vi "Log_MessageHandler_AddMessageToLog.vi"(7 "EVE reference in":refnum<data-value>, 8 "error in (no error)":errorcluster, 10 "Messages.lvclass":refnum<class "Messages.lvclass">, 11 "MessageHandler.lvclass in":refnum<class "MessageHandler.lvclass">) -> (0 "error out":errorcluster, 3 "MessageHandler.lvclass out":refnum<class "MessageHandler.lvclass">)   [LabVIEW 2013, in "MessageHandler.lvclass"]
uses:
  Class/MessageHandler.lvclass
  001 - MAIN/Class/Messages/Messages.lvclass
  001 - MAIN/Class/EVE/EVE.lvclass
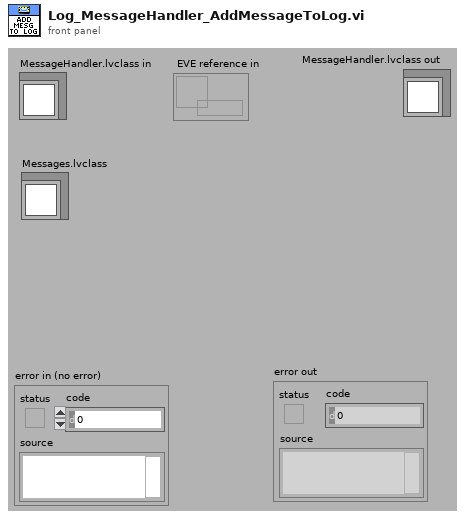
[diagram p1: front panel]
types:
  T1 = typedef "EVE.lvclass/App_GenericSettings.ctl" = cluster{"SpecificSettings":cluster{"FolderPath":path, "XMLFile":string}, "Log":cluster{"MaxLogFiles":i32, "MaxLogMessagesPerFile":i32}, "Debug":cluster{"Active":bool}, "Dictionnary":cluster{"FolderPath":path, "TradFile":string}, "Ressources":cluster{"FolderPath":path}}
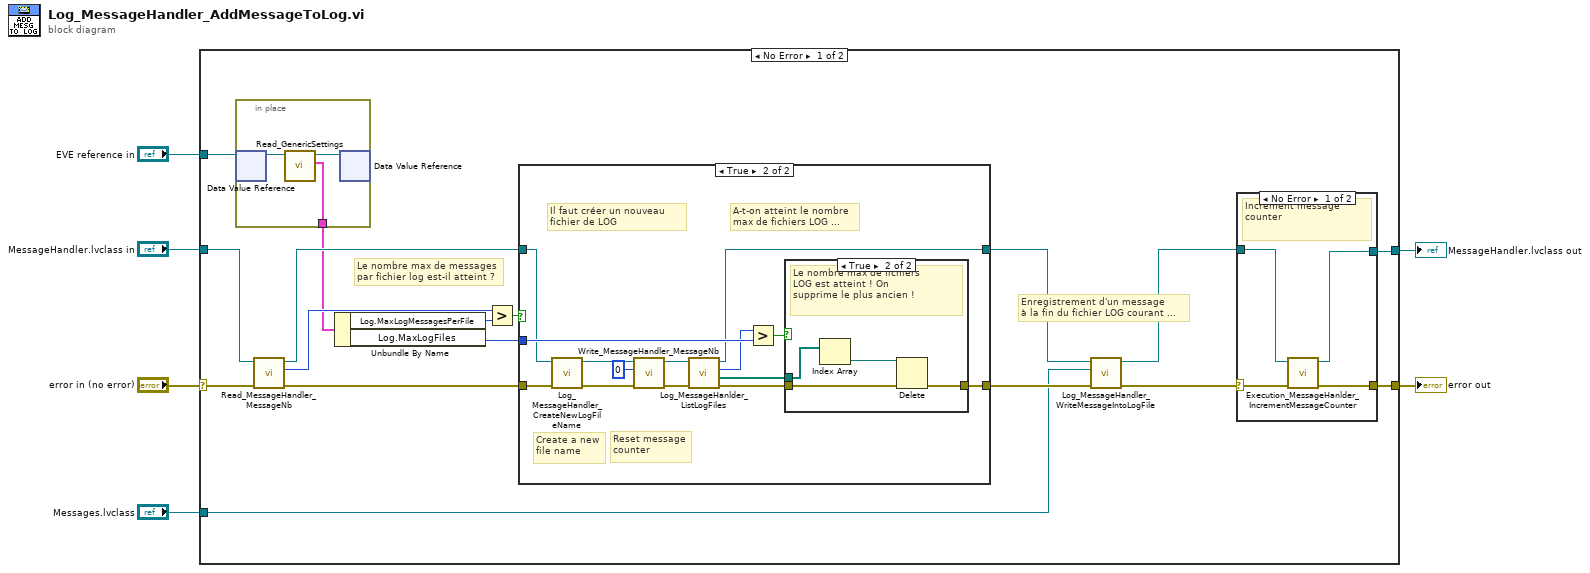
[diagram p0: block diagram]
diagram:
  n1 = case shown="No Error" "error in (no error)" {
    selector: "error in (no error)" -> [w18 w55]
    tunnel: [w20 w55] -> w5
    tunnel: "MessageHandler.lvclass in" -> [w15 w54]
    tunnel: [w19 w54] -> w3
    tunnel: "Messages.lvclass" -> [w10 _]
    tunnel: "EVE reference in" -> [w9 _]
    frame No Error {
      # "Enregistrement d'un message\nà la fin du fichier LOG courant ..."
      # "Le nombre max de messages\npar fichier log est-il atteint ?"
      n2 = in-place {
        in-place-border: [w24] -> w8
        n3 = in-place-dvr #1(w9) -> (w26:refnum<class "EVE.lvclass">)  [unwired: 1 out]
        n4 = call-dynamic "Read_GenericSettings.vi"("EVE in"=w26) -> ("GenericSettings"=w24:T1, "EVE out"=w25:refnum<class "EVE.lvclass">)  [unwired: 8 in, 1 out]
        n5 = in-place-dvr #1(w25) -> ()  [unwired: 2 out]
      }
      n6 = call-dynamic "Read_MessageHandler_MessageNb.vi"("error in (no error)"=w18, "MessageHandler in"=w15) -> ("error out"=w7:errorcluster, "Message number"=w17:u32, "MessageHandler out"=w16:refnum<class "MessageHandler.lvclass">)  [unwired: 7 in]
      n7 = Unbundle By Name(w8) -> ("Log.MaxLogMessagesPerFile"=w23:i32, "Log.MaxLogFiles"=w21:i32)
      n8 = Greater?(x=w17, y=w23) -> (0:w22:bool)
      n9 = case shown="True" w22 {
        tunnel: w7 -> [w33 w45]
        tunnel: w16 -> [w34 w44]
        tunnel: [w34 w37] -> w13
        tunnel: [w33 w46] -> w14
        tunnel: w21 -> [_ w48]
        frame False {
          # "Le nombre max de messages\npar fichier n'est pas encore\natteint !"
        }
        frame True {
          # "Reset message\ncounter"
          # "Create a new\nfile name"
          # "A-t-on atteint le nombre\nmax de fichiers LOG ..."
          # "Il faut créer un nouveau\nfichier de LOG"
          n10 = call-dynamic "Log_MessageHandler_CreateNewLogFileName.vi"("error in (no error)"=w45, "MessageHandler in"=w44) -> ("error out"=w43:errorcluster, "MessageHandler out"=w42:refnum<class "MessageHandler.lvclass">)  [unwired: 8 in]
          n11 = call-dynamic "Write_MessageHandler_MessageNb.vi"("error in (no error)"=w43, "Message number"=u32 0, "MessageHandler in"=w42) -> ("error out"=w40:errorcluster, "MessageHandler out"=w38:refnum<class "MessageHandler.lvclass">)  [unwired: 7 in]
          n12 = call-dynamic "Log_MessageHanlder_ListLogFiles.vi"("error in (no error)"=w40, "MessageHandler in"=w38) -> ("error out"=w39:errorcluster, "Log file paths"=w35:path[], "Log file nb"=w36:u32, "MessageHandler out"=w37:refnum<class "MessageHandler.lvclass">)  [unwired: 6 in]
          n13 = Greater?(x=w36, y=w48) -> (0:w47:bool)
          n14 = case shown="True" w47 {
            tunnel: w39 -> [w49 w52]
            tunnel: w35 -> [_ w53]
            tunnel: [w49 w51] -> w46
            frame False {
              # "Le nombre max de fichiers\nn'est pas atteint !"
            }
            frame True {
              # "Le nombre max de fichiers\nLOG est atteint ! On \nsupprime le plus ancien !"
              n15 = Index Array(array=w53) -> (element=w50:path)  [unwired: 1 in]
              n16 = Delete(path (use dialog)=w50, error in=w52) -> (error out=w51:errorcluster)  [unwired: 3 in, 2 out]
            }
          }
        }
      }
      n17 = call-dynamic "Log_MessageHandler_WriteMessageIntoLogFile.vi"("error in (no error)"=w14, "Messages.lvclass"=w10, "MessageHandler in"=w13) -> ("error out"=w11:errorcluster, "MessageHandler out"=w12:refnum<class "MessageHandler.lvclass">)  [unwired: 7 in]
      n18 = case shown="No Error" w11 {
        selector: w11 -> [w28 w31]
        tunnel: w12 -> [w30 w32]
        tunnel: [w27 w31] -> w20
        tunnel: [w29 w32] -> w19
        frame No Error {
          # "Increment message counter"
          n19 = call-dynamic "Execution_MessageHanlder_IncrementMessageCounter.vi"("error in (no error)"=w28, "MessageHandler in"=w30) -> ("error out"=w27:errorcluster, "MessageHandler out"=w29:refnum<class "MessageHandler.lvclass">)  [unwired: 8 in]
        }
        frame Error {
        }
      }
    }
    frame Error {
    }
  }
  "error out" <- w5
  "MessageHandler.lvclass out" <- w3
